vi "LVFunction_Imop_Check_ClosedLoopSecurity_Custom.vi"(0 "CorrectionDataManager":refnum<class "CorrectionDataManager.lvclass">, 5 "ClosedLoopSecurity":T2, 7 "CurrentPosition":T3, 9 "DeltaPosition":T3, 11 "error IO":errorcluster, 12 "HasoSlopes in":refnum<class "HasoSlopes.lvclass">, 13 "Fill Percent":sgl) -> (6 "ClosedLoopSecurityActivationParams":T1, 15 "error IO out":errorcluster)   [LabVIEW 2020]
doc: "Compute slopes from modal coefficients that represent them in a given basis of\npolynomials provided by ComputePhaseSet.\n\n--------------------------------------------------------------------------------\n\nTypePhaseIn\n TypePhase Polynomial bases enumeration.\n\nTypePhaseOut\n TypePhase Polynomial bases enumeration.\n\nslopes\n cHasoSlopes object.\n\nComputePhaseSet\n cComputePhaseSet object.\n\ncoefs\n cModalCoef object.\n\nErrorIn\n Error\nErrorOut\n Error"
uses:
  CorrectionDataManager.lvclass
  Wavefront Corrector Position.ctl
  HasoSlopes.lvclass
  ClosedLoopSecurityActivation.lvclass
  ClosedLoopSecurity.lvclass
  ClosedLoopSecurityActivationResults.ctl
  LVClass_HasoSlopes Read HasoSlopes _ property.vi
  LVClass_CorrectionDataManager Read CorrectionDataManager.vi
  LVClass_ClosedLoopSecurity Read ClosedLoopSecurity.vi
  LVClass_ClosedLoopSecurityActivation Read ClosedLoopSecurityActivation ptr.vi
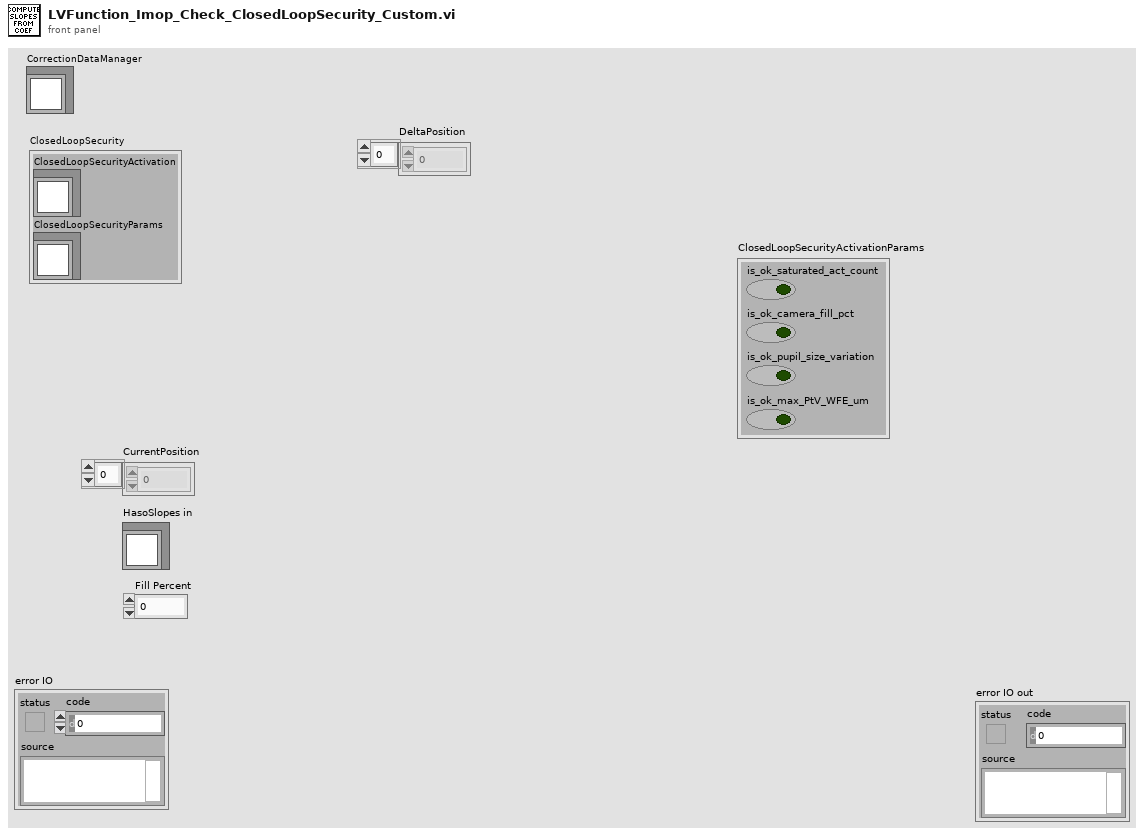
[diagram p1: front panel]
types:
  T1 = typedef "ClosedLoopSecurityActivationResults.ctl" = cluster{"is_ok_saturated_act_count":bool, "is_ok_camera_fill_pct":bool, "is_ok_pupil_size_variation":bool, "is_ok_max_PtV_WFE_um":bool}
  T2 = cluster{"ClosedLoopSecurityActivation":refnum<class "ClosedLoopSecurityActivation.lvclass">, "ClosedLoopSecurityParams":refnum<class "ClosedLoopSecurity.lvclass">}
  T3 = typedef "Wavefront Corrector Position.ctl" = sgl[]
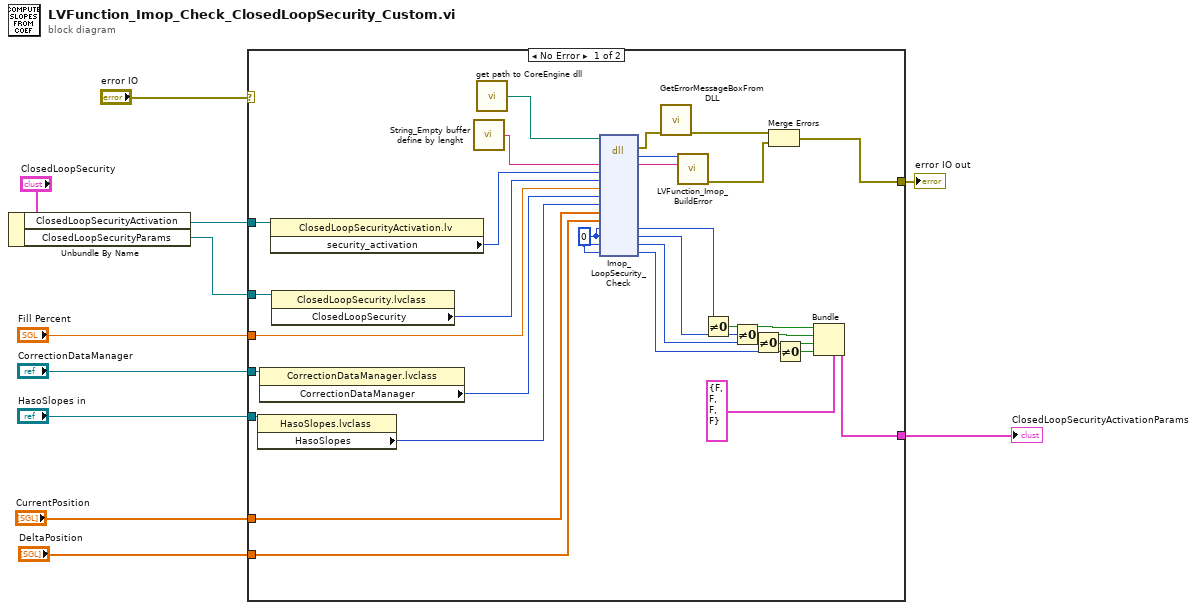
[diagram p0: block diagram]
diagram:
  n1 = Unbundle By Name("ClosedLoopSecurity") -> ("ClosedLoopSecurityActivation"=w5:refnum<class "ClosedLoopSecurityActivation.lvclass">, "ClosedLoopSecurityParams"=w4:refnum<class "ClosedLoopSecurity.lvclass">)
  n2 = case shown="No Error" "error IO" {
    selector: "error IO" -> [_ w42]
    tunnel: [w34 w42] -> w10
    tunnel: w5 -> [w33 _]
    tunnel: w4 -> [w32 _]
    tunnel: "CorrectionDataManager" -> [w31 _]
    tunnel: "Fill Percent" -> [w27 _]
    tunnel: "HasoSlopes in" -> [w30 _]
    tunnel: "CurrentPosition" -> [w13 _]
    tunnel: "DeltaPosition" -> [w24 _]
    tunnel: [w15 _] -> w1
    frame No Error {
      w12 = u8 0 ("is_ok_saturated_act_count")
      n3 = property class="HasoSlopes.lvclass"(reference=w30) -> ("HasoSlopes"=w25:i32)  [unwired: 1 in, 2 out]
      n4 = property class="CorrectionDataManager.lvclass"(reference=w31) -> ("CorrectionDataManager"=w26:i32)  [unwired: 1 in, 2 out]
      n5 = property class="ClosedLoopSecurityActivation.lv"(reference=w33) -> ("security_activation"=w29:i32)  [unwired: 1 in, 2 out]
      n6 = property class="ClosedLoopSecurity.lvclass"(reference=w32) -> ("ClosedLoopSecurity"=w28:i32)  [unwired: 1 in, 2 out]
      n7 = call "String_Empty buffer define by lenght.vi"() -> ("Empty buffer"=w39:string)  [unwired: 1 in]
      n8 = call "get path to CoreEngine dll.vi"() -> ("path to c_interface_vc100.dll"=w38:path)  [unwired: 12 in, 3 out]
      n9 = dll-call lib="D:/soft/HASO_v3/SVN_trunk/ImOpCoreEngine4_LV2011/DLLs/c_interface_vc100.dll" fn="Imop_LoopSecurity_Check"(path in=w38, "message"=w39, "security_activation"=w29, "security_params"=w28, "camera_fill_percentage"=w27, "correction_data_manager"=w26, "delta_slopes_pupil"=w25, "CurrentPosition"=w13, "delta_commands"=w24, "is_ok_saturated_act_count"=w12, "is_ok_camera_fill_pct"=w12, "is_ok_pupil_size_variation"=w12, "is_ok_loop_gain"=w12) -> (error out=w37:errorcluster, "return type"=w41:i32, "message"=w40:string, "is_ok_saturated_act_count"=w19:u8, "is_ok_camera_fill_pct"=w18:u8, "is_ok_pupil_size_variation"=w17:u8, "is_ok_loop_gain"=w16:u8)  [unwired: 9 in, 1 out]
      n10 = call "GetErrorMessageBoxFromDLL.vi"("error IN"=w37) -> ("error OUT"=w36:errorcluster)  [unwired: 10 in]
      n11 = call "LVFunction_Imop_BuildError.vi"("code"=w41, "String to Prepend to source (\"\")"=w40) -> ("error out"=w35:errorcluster)  [unwired: 13 in]
      n12 = Not Equal To 0?(x=w19) -> (x != 0?=w23:bool)
      n13 = Not Equal To 0?(x=w18) -> (x != 0?=w22:bool)
      n14 = Not Equal To 0?(x=w17) -> (x != 0?=w21:bool)
      n15 = Merge Errors(w36, w35) -> (w34:errorcluster)
      n16 = Not Equal To 0?(x=w16) -> (x != 0?=w20:bool)
      n17 = Bundle(cluster=T1 {"is_ok_saturated_act_count"=FALSE, "is_ok_camera_fill_pct"=FALSE, "is_ok_pupil_size_variation"=FALSE, "is_ok_max_PtV_WFE_um"=FALSE} ("ClosedLoopSecurityActivationParams"), "is_ok_saturated_act_count"=w23, "is_ok_camera_fill_pct"=w22, "is_ok_pupil_size_variation"=w21, "is_ok_max_PtV_WFE_um"=w20) -> (w15:T1)
    }
    frame Error {
    }
  }
  "error IO out" <- w10
  "ClosedLoopSecurityActivationParams" <- w1
